vi "SPI_Read - Copy.vi"(0 "bit_index":i32, 3 "rising_edge":bool) -> (9 "SDI":bool)   [LabVIEW 2019]
doc: "This Vi Read a slave message based on SPI protocol. It works with a clock handler and inside a loop"
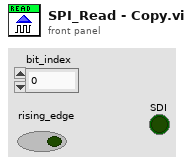
[diagram p1: front panel]
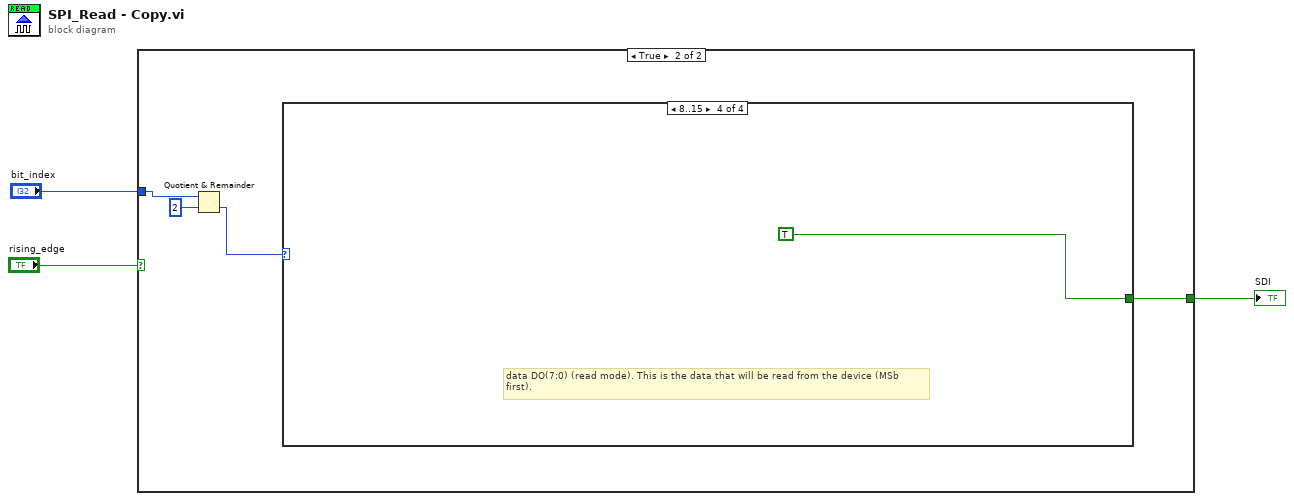
[diagram p0: block diagram]
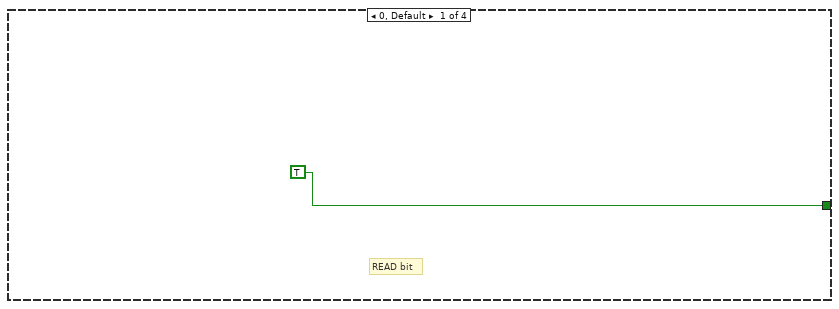
[diagram p3: hidden frame]
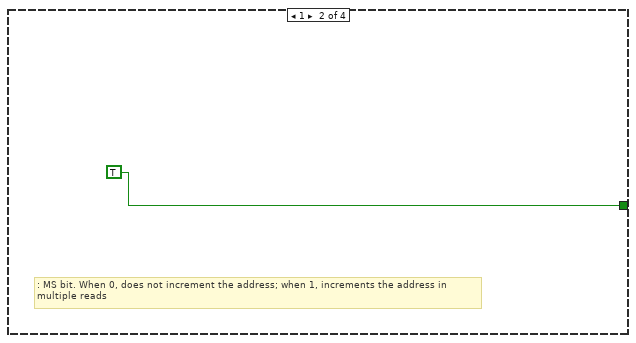
[diagram p4: hidden frame]
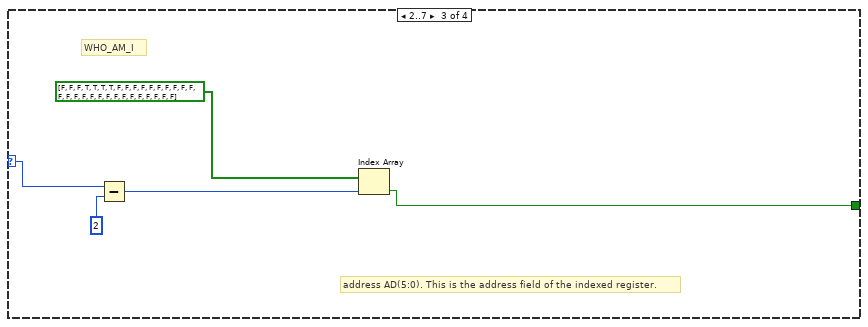
[diagram p5: hidden frame]
diagram:
  n1 = case shown="True" "rising_edge" {
    tunnel: "bit_index" -> [_ w6]
    tunnel: [_ w7] -> w1
    frame False {
    }
    frame True {
      n2 = Quotient & Remainder(x=w6, y=2) -> (floor(x/y)=w4:i32)  [unwired: 1 out]
      n3 = case shown="8..15" w4 {
        selector: w4 -> [_ _ w14 _]
        tunnel: [TRUE TRUE w10 TRUE ("SDO_Msg")] -> w7
        frame 0, Default {
          # "READ bit"
        }
        frame 1 {
          # ": MS bit. When 0, does not increment the address; when 1, increments the address in\nmultiple reads"
        }
        frame 2..7 {
          # "address AD(5:0). This is the address field of the indexed register."
          # "WHO_AM_I"
          n4 = Subtract(x=w14, y=2) -> (x-y=w12:i32)
          n5 = Index Array(array=bool[] [FALSE, FALSE, FALSE, TRUE, TRUE, TRUE, TRUE, FALSE, FALSE, FALSE, FALSE, FALSE, FALSE, FALSE, FALSE, FALSE, FALSE, FALSE, FALSE, FALSE, FALSE, FALSE, FALSE, FALSE, FALSE, FALSE, FALSE, FALSE, FALSE, FALSE, FALSE, FALSE], index=w12) -> (element=w10:bool)
        }
        frame 8..15 {
          # "data DO(7:0) (read mode). This is the data that will be read from the device (MSb\nfirst)."
        }
      }
    }
  }
  "SDI" <- w1
